vi "buttons.vi"() -> ()   [LabVIEW 2017]
doc: "collection of buttons"
panel:
  out "Boolean 6":bool
  out "Boolean":bool
  out "Boolean 5":bool
  out "Boolean 4":bool
  out "Boolean 3":bool
  out "Boolean 2":bool
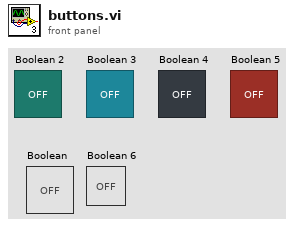
[diagram p1: front panel]
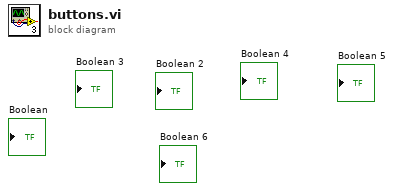
[diagram p0: block diagram]
diagram:
